vi "IsSatisfied.vi"(10 "Product":refnum<class "Product.lvclass">, 11 "ColorSpecification":refnum<class "ColorSpecification.lvclass">) -> (2 "IsSatisfied":bool)   [LabVIEW 2018, in "ColorSpecification.lvclass"]
uses:
  ColorSpecification.lvclass
  Product/Product.lvclass
  ColorSpecification.lvclass/ColorSpecification.ctl
  Product/Product.lvclass/Product.ctl
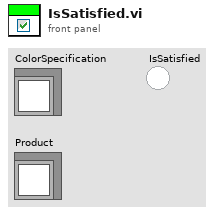
[diagram p1: front panel]
types:
  T1 = typedef "Product.lvclass/Color.ctl" = enum16{"Blue", "Green", "Red"}
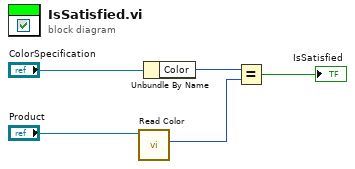
[diagram p0: block diagram]
diagram:
  n1 = call "Read Color.vi"("Product In"="Product") -> ("Color"=w2:T1)  [unwired: 9 in, 1 out]
  n2 = Unbundle By Name("ColorSpecification") -> ("Color"=w3:T1)
  n3 = Equal?(x=w3, y=w2) -> (x = y?=→"IsSatisfied":bool)
